vi "Main.vi"() -> ()   [LabVIEW 2013]
uses:
  <userlib>/labvvis/New Image/New Image (Grey).vi
  <userlib>/labvvis/labvvis.lvlib
panel:
  in  "stop":bool
  in  "?":bool
  out "rock":u8
  out "scissor_column_counter":u8
  out "paper_colum_counter":u8
  out "scissor":bool
  out "paper":bool
  out "Rock":bool
  out "Error":string
  out "Input Hand Gesture":picture
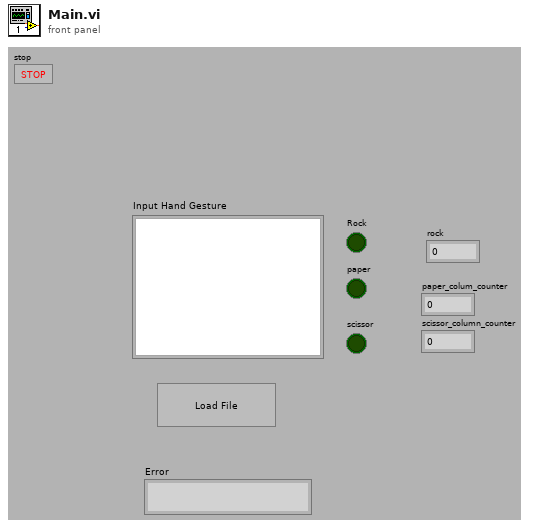
[diagram p1: front panel]
types:
  T1 = typedef "imagedata.ctl" = cluster{"image type":i32, "image depth":i32, "image":u8[], "mask":u8[], "colors":u32[], "Rectangle":cluster{"left":i16, "top":i16, "right":i16, "bottom":i16}}
  T2 = typedef "labvvis.lvlib/VVIS Image.ctl" = cluster{"Image ID":i16, "Channel ID":i16}
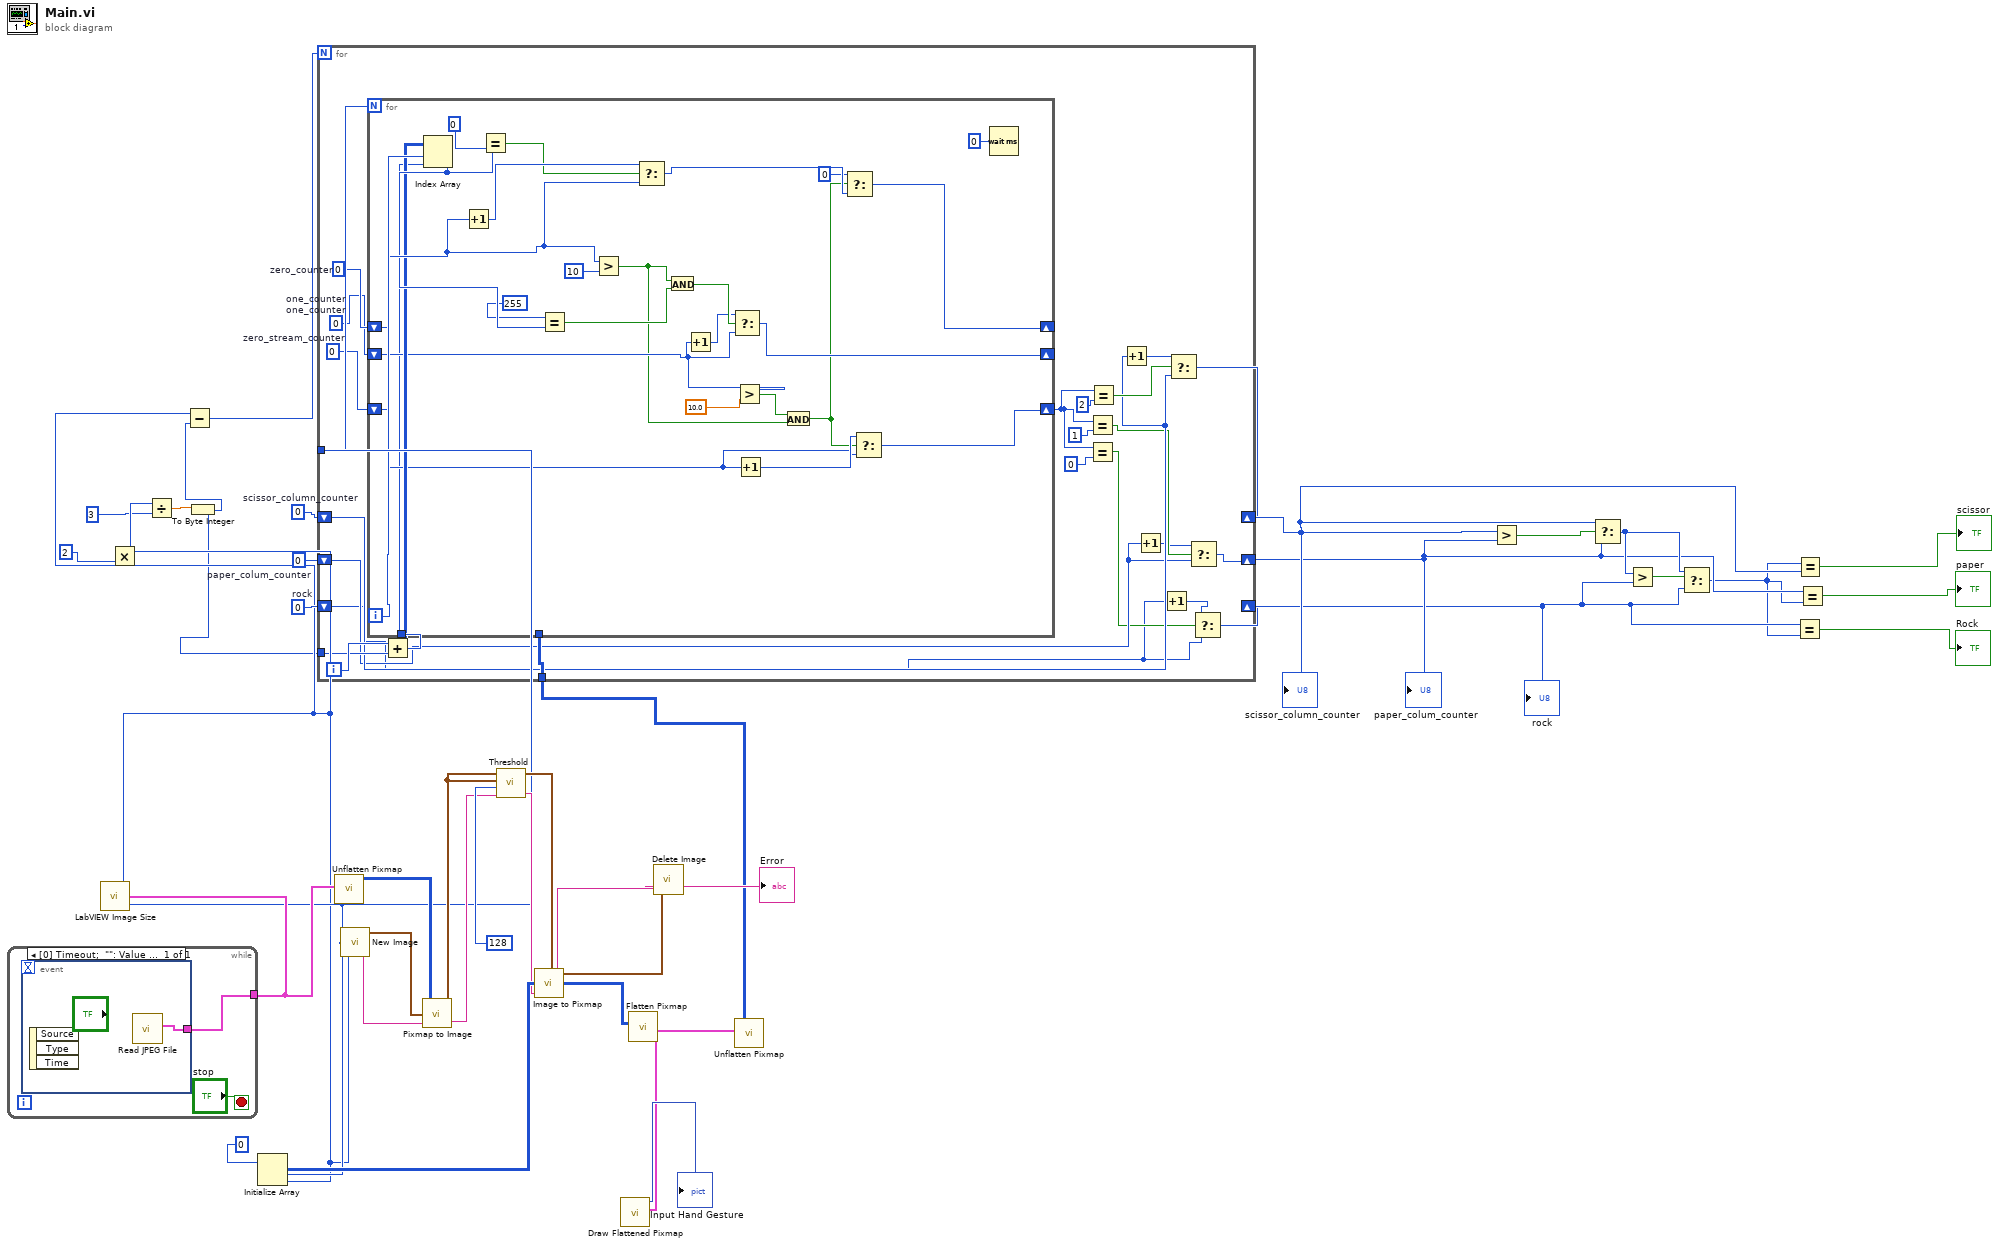
[diagram p0: block diagram]
diagram:
  w14 = u8 0  # rock
  w15 = u8 0  # paper_colum_counter
  w16 = u8 0  # scissor_column_counter
  n1 = while {
    tunnel: [w41] -> w27
    stop <- "stop" stop-if-true
    n2 = event shown="[0] Timeout;  \"\": Value Change" {
      selector: _ -> [_]
      dyn-events: _ -> [_]
      timeout: _ -> [_]
      tunnel: [w42] -> w41
      event Timeout; Value Change {
        n3 = event-data() -> ()  [unwired: 1 in, 3 out]
        n4 = call <vilib>:"Read JPEG File.vi"() -> ("image data"=w42:T1)  [unwired: 9 in, 2 out]
      }
    }
  }
  n5 = call <userlib>:"LabVIEW Image Size.vi"("Cluster"=w27) -> ("Width"=w13:i16, "Height"=w24:i16)
  n6 = Multiply(x=w13, y=i16 2) -> (x*y=w19:i16)
  n7 = Divide(x=w19, y=i16 3) -> (x/y=w12:dbl)
  n8 = To Byte Integer(number=w12) -> (8bit integer=w11:i8)
  n9 = Subtract(x=w13, y=w11) -> (x-y=w17:i16)
  n10 = Initialize Array(0, w24, w13) -> (w32:i32[][])
  n11 = call <vilib>:"Unflatten Pixmap.vi"("image data"=w27) -> ("24-bit pixmap"=w35:u32[][])  [unwired: 4 in, 6 out]
  n12 = call-poly <userlib>:"New Image.vi"("Height"=w24, "Width"=w13) -> ("Error"=w28:string, "VVIS Image"=w36:T2)  [unwired: 2 in]
  n13 = call <userlib>:"Pixmap to Image.vi"("Error"=w28, "Output Image"=w36, "Input Pixmap"=w35) -> ("Error"=w34:string, "Output Image"=w33:T2)
  n14 = call <userlib>:"Threshold.vi"("Error"=w34, "Threshold"=i16 128, "Output Image"=w33, "Input Image"=w33) -> ("Error"=w31:string, "Input Image"=w25:T2)  [unwired: 1 out]
  n15 = call <userlib>:"Image to Pixmap.vi"("Error"=w31, "Output Pixmap"=w32, "Image"=w25) -> ("Error"=w30:string, "Output Pixmap"=w22:u32[][], "Image"=w26:T2)
  n16 = call <vilib>:"Flatten Pixmap.vi"("8-bit pixmap"=w22) -> ("image data"=w23:T1)  [unwired: 10 in]
  n17 = call <vilib>:"Draw Flattened Pixmap.vi"("image data"=w23) -> ("new picture"=→"Input Hand Gesture":picture)  [unwired: 8 in]
  n18 = call <userlib>:"Delete Image.vi"("Error"=w30, "Image"=w26) -> ("Error"=→"Error":string)  [unwired: 1 in]
  n19 = call <vilib>:"Unflatten Pixmap.vi"("image data"=w23) -> ("8-bit pixmap"=w21:u8[][])  [unwired: 4 in, 6 out]
  n20 = for {
    N: w17 -> [_]
    tunnel: w24 -> [w66]
    tunnel: w21 -> [w65]
    tunnel: w11 -> [w63]
    shift-right: [w51] -> w7
    shift-left: w16 -> [w53]
    shift-right: [w47] -> w5
    shift-left: w15 -> [w49]
    shift-right: [w43] -> w3
    shift-left: w14 -> [w45]
    i -> [w64]
    w59 = 0  # zero_stream_counter
    w60 = u8 0  # one_counter one_counter
    w61 = u8 0  # zero_counter
    n21 = Add(x=w64, y=w63) -> (x+y=w62:i32)
    n22 = for {
      N: w66 -> [_]
      tunnel: w65 -> [w84]
      tunnel: w62 -> [w67]
      shift-right: [w71] -> _
      shift-left: w61 -> [w89]
      shift-right: [w81] -> _
      shift-left: w60 -> [w79]
      shift-right: [w76] -> w58
      shift-left: w59 -> [w77]
      i -> [w92]
      n23 = Index Array(array=w84, index (row)=w92, index (col)=w67) -> (element=w87:u8)
      n24 = Increment(x=w89) -> (x+1=w90:u8)
      n25 = Equal?(x=w87, y=u8 0) -> (x = y?=w69:bool)
      n26 = Equal?(x=u8 255, y=w87) -> (x = y?=w85:bool)
      n27 = Greater?(x=w89, y=u8 10) -> (0:w74:bool)
      n28 = Select(t=w90, s=w69, f=w89) -> (s? t:f=w73:u8)
      n29 = And(x=w74, y=w85) -> (x .and. y?=w83:bool)
      n30 = Increment(x=w79) -> (x+1=w82:u8)
      n31 = Select(t=w82, s=w83, f=w79) -> (s? t:f=w81:u8)
      n32 = Greater?(x=w79, y=10.0) -> (0:w75:bool)
      n33 = Increment(x=w77) -> (x+1=w78:i32)
      n34 = And(x=w75, y=w74) -> (x .and. y?=w68:bool)
      n35 = Select(t=u8 0, s=w68, f=w73) -> (s? t:f=w71:u8)
      n36 = Select(t=w78, s=w68, f=w77) -> (s? t:f=w76:i32)
      n37 = Wait (ms)(milliseconds to wait=u32 0) -> ()  [unwired: 1 out]
    }
    n38 = Equal?(x=w58, y=1) -> (x = y?=w50:bool)
    n39 = Equal?(x=w58, y=0) -> (x = y?=w46:bool)
    n40 = Equal?(x=w58, y=2) -> (x = y?=w54:bool)
    n41 = Increment(x=w53) -> (x+1=w52:u8)
    n42 = Increment(x=w49) -> (x+1=w48:u8)
    n43 = Increment(x=w45) -> (x+1=w44:u8)
    n44 = Select(t=w52, s=w54, f=w53) -> (s? t:f=w51:u8)
    n45 = Select(t=w48, s=w50, f=w49) -> (s? t:f=w47:u8)
    n46 = Select(t=w44, s=w46, f=w45) -> (s? t:f=w43:u8)
  }
  "paper_colum_counter" <- w5
  "scissor_column_counter" <- w7
  "rock" <- w3
  n47 = Greater?(x=w7, y=w5) -> (0:w10:bool)
  n48 = Select(t=w7, s=w10, f=w5) -> (s? t:f=w9:u8)
  n49 = Greater?(x=w9, y=w3) -> (0:w8:bool)
  n50 = Select(t=w9, s=w8, f=w3) -> (s? t:f=w2:u8)
  n51 = Equal?(x=w3, y=w2) -> (x = y?=→"Rock":bool)
  n52 = Equal?(x=w2, y=w7) -> (x = y?=→"scissor":bool)
  n53 = Equal?(x=w5, y=w2) -> (x = y?=→"paper":bool)
